vi "Configure Source to Sequence-Ganging.vi"(8 "error in":errorcluster, 11 "Source to seq config - Ganging":T4={"Source Ganged Session Out"={"Ganged Config"=enum."Series", "Session List"=[], "Session Mode"=[], "Channel"=[]}, "Source sweep values"=[], "Load sweep points"=0, "Source output function"=1006, "Source transient response"=1038, "Source voltage/current gain bandwidth"=0.0, "Source voltage/current compensation frequency"=0.0, "Source voltage/current pole-zero ratio"=0.0, "Source aperture time"=0.0, "Source source delay"=0.0} {"Source transient response" items=["Slow"=1041, "Normal"=1038, "Fast"=1039, "Custom"=1042]; "Source output function" items=["DC Voltage"=1006, "DC Current"=1007, "Pulse Voltage"=1049, "Pulse Current"=1050]; "Source sweep values" format="%#_13g"}) -> (0 "error out":errorcluster, 3 "Ganged Session Out":T1)   [LabVIEW 2021]
doc: "This vi configures the source to sequence."
uses:
  controls/Source to Sequence Config-Ganging.ctl
  channel ganging/shared subVIs/ctl/NIDCPower_channel_ganging - ctl - ganged config.ctl
  channel ganging/shared subVIs/ctl/NIDCPower_channel_ganging - ctl - channel mode.ctl
  channel ganging/shared subVIs/ctl/NIDCPower_channel_ganging - ctl - ganged session.ctl
  <instrlib>/niDCPower/nidcpower.llb/niDCPower Source Mode.ctl
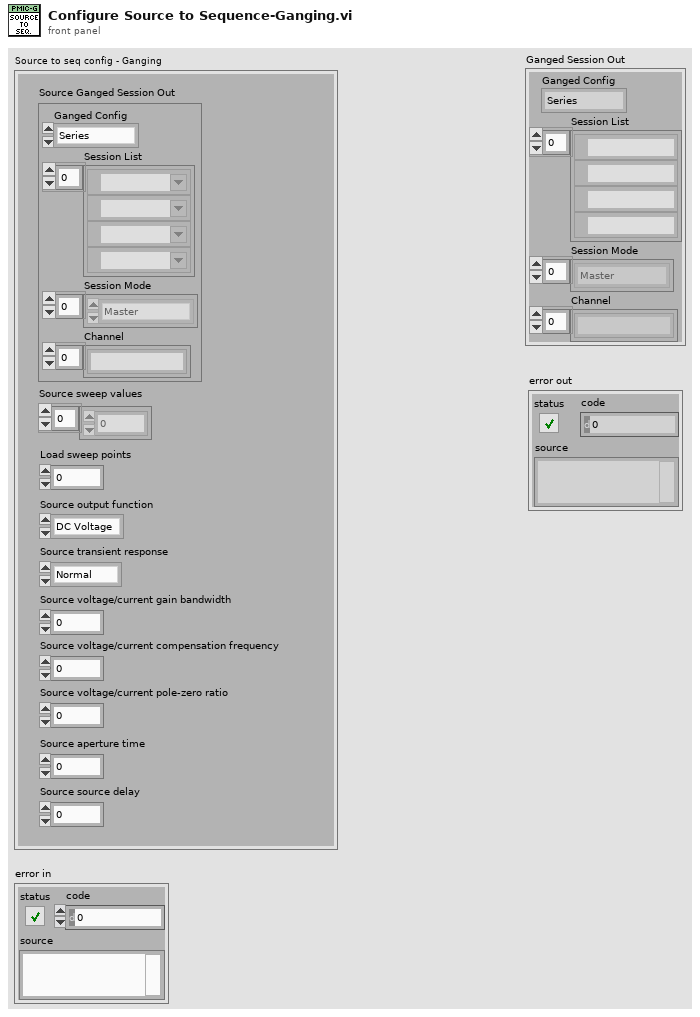
[diagram p1: front panel]
types:
  T1 = typedef "NIDCPower_channel_ganging - ctl - ganged session.ctl" = cluster{"Ganged Config":T2, "Session List":refnum<k15>[], "Session Mode":T3[], "Channel":string[]}
  T2 = typedef "NIDCPower_channel_ganging - ctl - ganged config.ctl" = enum32{"Series", "Parallel", "Manual"}
  T3 = typedef "NIDCPower_channel_ganging - ctl - channel mode.ctl" = enum32{"Master", "Slave", "Slave - Inverted"}
  T4 = typedef "Source to Sequence Config-Ganging.ctl" = cluster{"Source Ganged Session Out":cluster{"Ganged Config":T2, "Session List":refnum<k15>[], "Session Mode":T3[], "Channel":string[]}, "Source sweep values":dbl[], "Load sweep points":i32, "Source output function":i32, "Source transient response":i32, "Source voltage/current gain bandwidth":dbl, "Source voltage/current compensation frequency":dbl, "Source voltage/current pole-zero ratio":dbl, "Source aperture time":dbl, "Source source delay":dbl}
  T5 = typedef "niDCPower Source Mode.ctl" = i32
  T6 = cluster{"Ganged Config":T2, "Session List":refnum<k15>[], "Session Mode":T3[], "Channel":string[]}
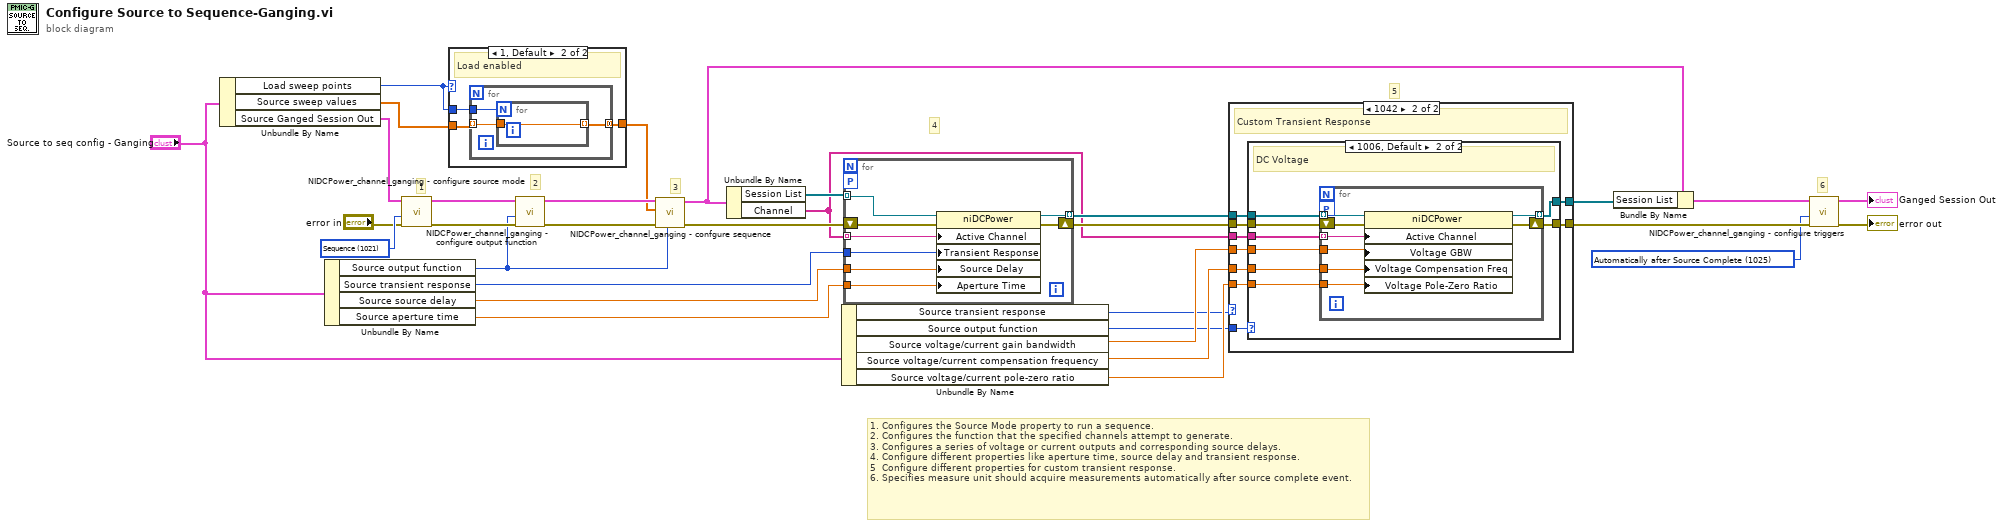
[diagram p0: block diagram]
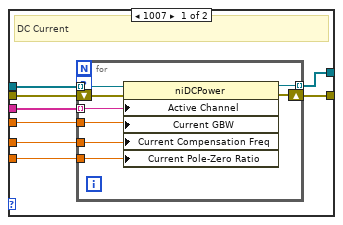
[diagram p3: hidden frame]
diagram:
  w6 = 1025 items=["Automatically after Source Complete"=1025, "On Demand"=1026, "On Measure Trigger"=1027] ("Measure When")
  w29 = T5 1021 items=["Single Point"=1020, "Sequence"=1021] ("source mode")
  # "6"
  # "5"
  # "4"
  # "3"
  # "2"
  # "1"
  # "1. Configures the Source Mode property to run a sequence.\n2. Configures the function that the specified channels attempt to generate.\n3. Configures a series of voltage or current outputs and corresponding source delays.\n4. Configure different properties like aperture time, source delay and transient response. \n5  Configure different properties for custom transient response.\n6. Specifies measure unit should acquire measurements automatically after source complete event."
  n1 = Unbundle By Name("Source to seq config - Ganging") -> ("Load sweep points"=w21:i32, "Source sweep values"=w23:dbl[], "Source Ganged Session Out"=w25:T6)
  n2 = Unbundle By Name("Source to seq config - Ganging") -> ("Source output function"=w16:i32, "Source transient response"=w9:i32, "Source source delay"=w22:dbl, "Source aperture time"=w5:dbl)
  n3 = call "NIDCPower_channel_ganging - configure source mode.vi"("error in (no error)"="error in", "source mode"=w29, "Ganged Session In"=w25) -> ("error out"=w30:errorcluster, "Ganged Session Out"=w31:T1)  [unwired: 7 in]
  n4 = case shown="1, Default" w21 {
    tunnel: [w33 w36] -> w24
    tunnel: w23 -> [w33 w35]
    tunnel: w21 -> [_ w34]
    frame 0 {
      # "Load disabled"
    }
    frame 1, Default {
      # "Load enabled"
      n5 = for {
        tunnel: w34 -> [w39]
        tunnel: w35 -> [w38] mode=indexing
        tunnel: [w37] -> w36 mode=concatenating
        n6 = for {
          N: w39 -> [_]
          tunnel: w38 -> [w40]
          tunnel: [w40] -> w37 mode=indexing
        }
      }
    }
  }
  n7 = call "NIDCPower_channel_ganging - configure output function.vi"("error in (no error)"=w30, "output function"=w16, "Ganged Session In"=w31) -> ("error out"=w27:errorcluster, "Ganged Session Out"=w28:T1)  [unwired: 7 in]
  n8 = call "NIDCPower_channel_ganging - confgure sequence.vi"("output function"=w16, "error in (no error)"=w27, "Values"=w24, "Ganged Session In"=w28) -> ("error out"=w26:errorcluster, "Ganged Session Out"=w11:T1)  [unwired: 6 in]
  n9 = Unbundle By Name(w11) -> ("Session List"=w32:refnum<k15>[], "Channel"=w17:string[])
  n10 = Unbundle By Name("Source to seq config - Ganging") -> ("Source transient response"=w4:i32, "Source output function"=w3:i32, "Source voltage/current gain bandwidth"=w15:dbl, "Source voltage/current compensation frequency"=w13:dbl, "Source voltage/current pole-zero ratio"=w14:dbl)
  n11 = for {
    tunnel: [w48] -> w18 mode=indexing
    shift-right: [w46] -> w20
    shift-left: w26 -> [w47]
    workers-P: _ -> [_]
    tunnel: w32 -> [w45] mode=indexing
    tunnel: w17 -> [w44] mode=indexing
    tunnel: w9 -> [w43]
    tunnel: w22 -> [w42]
    tunnel: w5 -> [w41]
    n12 = property class="niDCPower"(reference=w45, error in=w47, "Active Channel"=w44, "Transient Response"=w43, "Source Delay"=w42, "Aperture Time"=w41) -> (reference out=w48:refnum<k15>, error out=w46:errorcluster)
  }
  n13 = case shown="1042" w4 {
    tunnel: w20 -> [w50 w59]
    tunnel: [w50 w58] -> w19
    tunnel: w18 -> [w49 w57]
    tunnel: w17 -> [_ w56]
    tunnel: w3 -> [_ w55]
    tunnel: w15 -> [_ w54]
    tunnel: w14 -> [_ w53]
    tunnel: w13 -> [_ w52]
    tunnel: [w49 w51] -> w12
    frame Default {
      # "Slow, Noramal and Fast Transient Response"
    }
    frame 1042 {
      # "Custom Transient Response"
      n14 = case shown="1006, Default" w55 {
        tunnel: w59 -> [w67 w83]
        tunnel: [w66 w82] -> w58
        tunnel: w57 -> [w65 w81]
        tunnel: w56 -> [w63 w80]
        tunnel: w54 -> [w64 w79]
        tunnel: w53 -> [w61 w77]
        tunnel: w52 -> [w62 w78]
        tunnel: [w60 w76] -> w51
        frame 1007 {
          # "DC Current"
          n15 = for {
            workers-P: _ -> [_]
            shift-right: [w74] -> w66
            shift-left: w67 -> [w75]
            tunnel: w65 -> [w73] mode=indexing
            tunnel: [w72] -> w60 mode=indexing
            tunnel: w64 -> [w71]
            tunnel: w63 -> [w70] mode=indexing
            tunnel: w62 -> [w69]
            tunnel: w61 -> [w68]
            n16 = property class="niDCPower"(reference=w73, error in=w75, "Active Channel"=w70, "Current GBW"=w71, "Current Compensation Freq"=w69, "Current Pole-Zero Ratio"=w68) -> (reference out=w72:refnum<k15>, error out=w74:errorcluster)
          }
        }
        frame 1006, Default {
          # "DC Voltage"
          n17 = for {
            workers-P: _ -> [_]
            shift-right: [w84] -> w82
            shift-left: w83 -> [w91]
            tunnel: w81 -> [w90] mode=indexing
            tunnel: [w89] -> w76 mode=indexing
            tunnel: w80 -> [w88] mode=indexing
            tunnel: w79 -> [w87]
            tunnel: w78 -> [w86]
            tunnel: w77 -> [w85]
            n18 = property class="niDCPower"(reference=w90, error in=w91, "Active Channel"=w88, "Voltage GBW"=w87, "Voltage Compensation Freq"=w86, "Voltage Pole-Zero Ratio"=w85) -> (reference out=w89:refnum<k15>, error out=w84:errorcluster)
          }
        }
      }
    }
  }
  n19 = Bundle By Name(cluster=w11, "Session List"=w12) -> (w10:T1)
  n20 = call "NIDCPower_channel_ganging - configure triggers.vi"("error in (no error)"=w19, "Measure When"=w6, "Ganged Session In"=w10) -> ("error out"=→"error out":errorcluster, "Ganged Session Out"=→"Ganged Session Out":T1)  [unwired: 7 in]
